vi "testEmptyPath.vi"(8 "error in (no error)":errorcluster) -> (0 "error out":errorcluster)   [LabVIEW 2019, in "TestCaseTest.lvlib" / "Fact.lvlib"]
uses:
  Fact.lvlib
  TestCase/Fact/Fact.lvclass
  Assertion/Assertion.lvlib
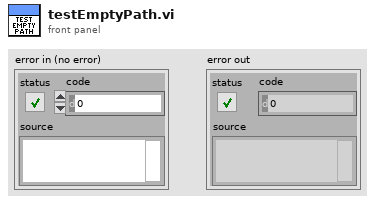
[diagram p1: front panel]
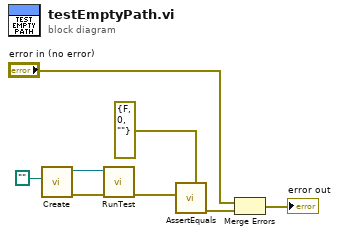
[diagram p0: block diagram]
diagram:
  n1 = call "Create.vi"("Path"=path "") -> ("error out"=w7:errorcluster, "Fact"=w8:refnum<class "Fact.lvclass">)  [unwired: 9 in]
  n2 = call-dynamic "RunTest.vi"("error in (no error)"=w7, "Fact in"=w8) -> ("error out"=w6:errorcluster)  [unwired: 8 in, 1 out]
  n3 = call "AssertEquals.vi"("Expected"=errorcluster {"status"=FALSE, "code"=0, "source"=""} ("error out"), "Actual"=w6) -> ("error out"=w4:errorcluster)  [unwired: 8 in, 1 out]
  n4 = Merge Errors("error in (no error)", w4) -> (→"error out":errorcluster)
